vi "Corr Transducers to Meas Header.vi"(8 "error in":errorcluster, 10 "measurement root path":path, 11 "transducers in":T2 {"channels"."Phase index" min=1 step=1}) -> (0 "error out":errorcluster, 2 "info data out":string, 3 "transducers out":T2 {"channels"."Phase index" min=1 step=1})   [LabVIEW 2020]
doc: "This VI will copy all transducer corrections to the measurement root path."
uses:
  Corr Tranducer Item.ctl
  octave/infolib/2D I64.vi
  octave/infolib/1D String.vi
  octave/infolib/1D I64.vi
  octave/infolib/infolib.lvlib
panel:
  # "ADC:"
  # "ADC:"
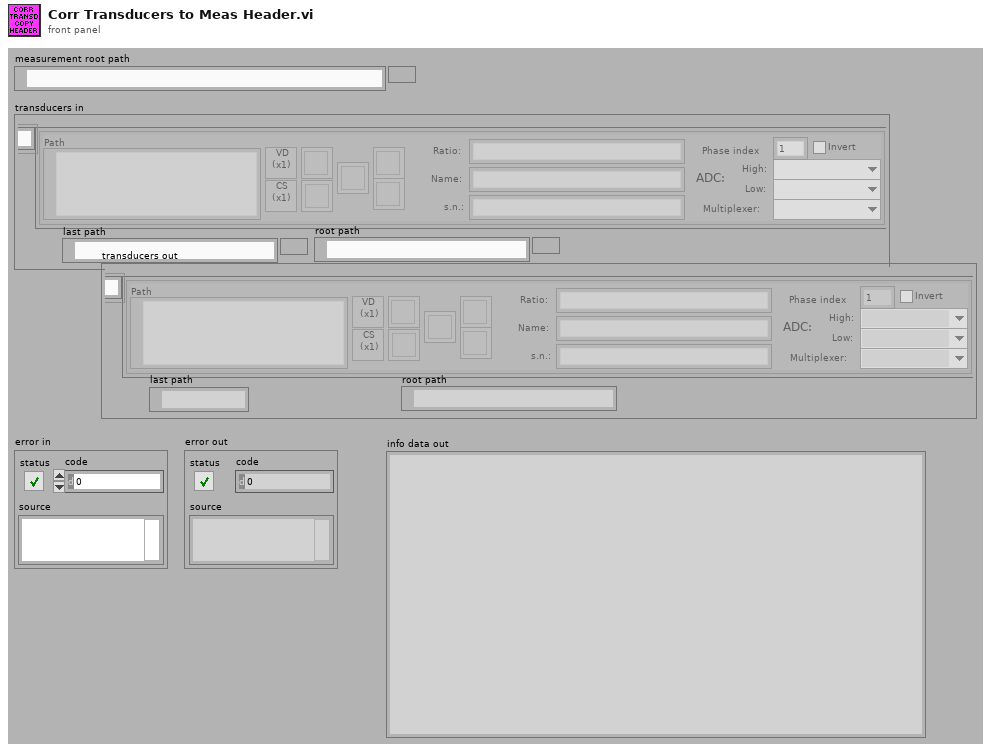
[diagram p1: front panel]
types:
  T1 = typedef "Corr Tranducer Item.ctl" = cluster{"Path":path, "Ratio:":string, "Name:":string, "btn rem":bool, "btn up":bool, "btn down":bool, "s.n.:":string, "btn open":bool, "ratio o/i":dbl, "chn hi":u16, "chn lo":u16, "Phase index":i32, "btn edit":bool, "mpx chn":u16, "btn vdx1":bool, "btn csx1":bool, "invert":bool}
  T2 = cluster{"channels":T1[], "last path":path, "root path":path}
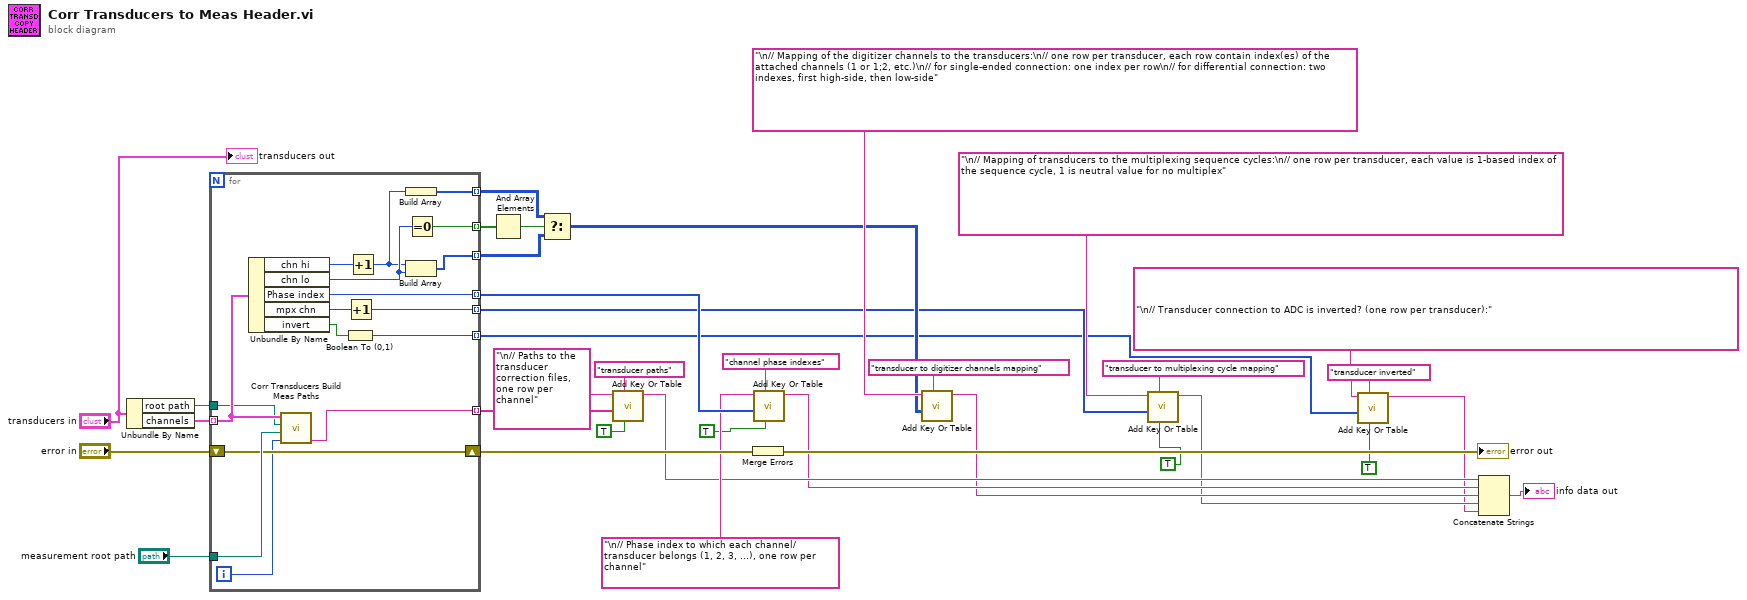
[diagram p0: block diagram]
diagram:
  n1 = Unbundle By Name("transducers in") -> ("root path"=w9:path, "channels"=w36:T1[])
  n2 = for {
    tunnel: w36 -> [w50] mode=indexing
    tunnel: "measurement root path" -> [w53]
    shift-right: [w52] -> w34
    shift-left: "error in" -> [w52]
    tunnel: [w51] -> w26 mode=indexing
    tunnel: [w49] -> w28 mode=indexing
    tunnel: [w46] -> w17 mode=indexing
    tunnel: [w44] -> w19 mode=indexing
    tunnel: [w42] -> w16 mode=indexing
    tunnel: [w40] -> w10 mode=indexing
    tunnel: w9 -> [w39]
    tunnel: [w37] -> w1 mode=indexing
    i -> [w47]
    n3 = Unbundle By Name(w50) -> ("chn hi"=w48:u16, "chn lo"=w45:u16, "Phase index"=w49:i32, "mpx chn"=w41:u16, "invert"=w38:bool)
    n4 = call "Corr Transducers Build Meas Paths.vi"("transducer index"=w47, "measurement folder root path"=w53, "transducer root path"=w39, "transducer"=w50) -> ("destination header realtive path"=w51:string)  [unwired: 3 out]
    n5 = Boolean To (0,1)(Boolean=w38) -> (0, 1=w37:i16)
    n6 = Increment(x=w41) -> (x+1=w40:u16)
    n7 = Increment(x=w48) -> (x+1=w43:u16)
    n8 = Build Array(w43) -> (w42:u16[])
    n9 = Build Array(w43, w45) -> (w46:u16[])
    n10 = Equal To 0?(x=w45) -> (x = 0?=w44:bool)
  }
  n11 = And Array Elements(Boolean array=w19) -> (logical AND=w18:bool)
  n12 = Select(t=w16, s=w18, f=w17) -> (s? t:f=w15:u16[][])
  n13 = call-poly "Add Key Or Table.vi"("collumn vector (F)"=TRUE ("column vector (F)"), "key description"="transducer paths", "string"=w26, "info data"="\n// Paths to the transducer correction files, one row per channel") -> ("info data out"=w22:string)  [unwired: 6 in, 1 out]
  n14 = Merge Errors(w34) -> (→"error out":errorcluster)
  n15 = call-poly "Add Key Or Table.vi"("collumn vector (F)"=TRUE ("column vector (F)"), "key description"="channel phase indexes", "numeric"=w28, "info data"="\n// Phase index to which each channel/transducer belongs (1, 2, 3, ...), one row per channel") -> ("info data out"=w21:string)  [unwired: 6 in, 1 out]
  n16 = call-poly "Add Key Or Table.vi"("key description"="transducer to digitizer channels mapping", "numeric"=w15, "info data"="\n// Mapping of the digitizer channels to the transducers:\n// one row per transducer, each row contain index(es) of the attached channels (1 or 1;2, etc.)\n// for single-ended connection: one index per row\n// for differential connection: two indexes, first high-side, then low-side") -> ("info data out"=w12:string)  [unwired: 8 in]
  n17 = call-poly "Add Key Or Table.vi"("collumn vector (F)"=TRUE ("column vector (F)"), "key description"="transducer to multiplexing cycle mapping", "numeric"=w10, "info data"="\n// Mapping of transducers to the multiplexing sequence cycles:\n// one row per transducer, each value is 1-based index of the sequence cycle, 1 is neutral value for no multiplex") -> ("info data out"=w11:string)  [unwired: 6 in, 1 out]
  n18 = call-poly "Add Key Or Table.vi"("collumn vector (F)"=TRUE ("column vector (F)"), "key description"="transducer inverted", "numeric"=w1, "info data"="\n// Transducer connection to ADC is inverted? (one row per transducer):") -> ("info data out"=w3:string)  [unwired: 6 in, 1 out]
  n19 = Concatenate Strings(w22, w21, w12, w11, w3) -> (→"info data out":string)
  "transducers out" <- "transducers in"
